vi "Clear Channel.vi"(8 "error in (no error)":errorcluster, 10 "Variant":variant, 11 "PI650 VoltageAmp in":refnum<class "PI650 VoltageAmp.lvclass">) -> (0 "error out":errorcluster, 3 "PI650 VoltageAmp out":refnum<class "PI650 VoltageAmp.lvclass">)   [LabVIEW 2020, in "Pickering.lvlib" / "PI650 VoltageAmp.lvclass"]
uses:
  PI650 VoltageAmp.lvclass
  PI650 VoltageAmp.lvclass/PI650 VoltageAmp.ctl
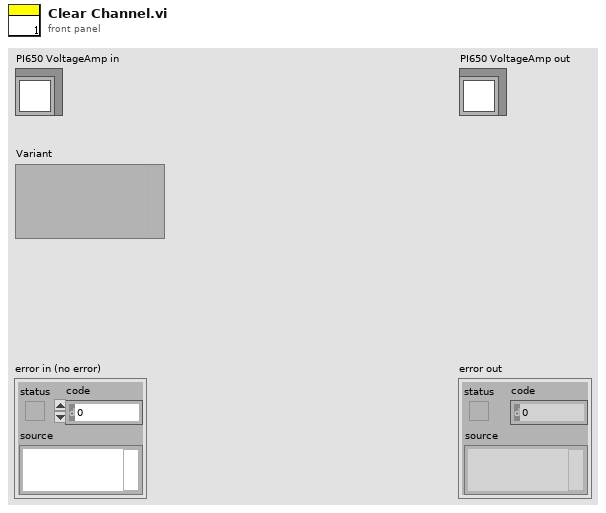
[diagram p1: front panel]
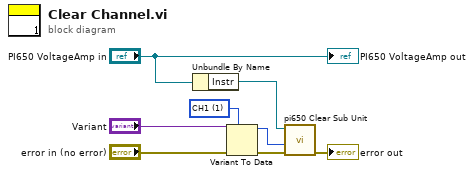
[diagram p0: block diagram]
diagram:
  w4 = u32 1 items=["CH1"=1, "CH2"=2, "CH3"=3, "CH4"=4, "CH5"=5] ("Channel (CH1)")
  n1 = Unbundle By Name("PI650 VoltageAmp in") -> ("Instr"=w7:refnum<visa-resource-name>)
  n2 = Variant To Data(error in="error in (no error)", type=w4, Variant="Variant") -> (data=w3:u32, error out=w2:errorcluster)
  n3 = call <instrlib>:"pi650 Clear Sub Unit.vi"("error in (no error)"=w2, "Subunit Number (6)"=w3, "instrument handle"=w7) -> ("error out"=→"error out":errorcluster)  [unwired: 7 in, 1 out]
  "PI650 VoltageAmp out" <- "PI650 VoltageAmp in"
